vi "Z900_navX_Util_DecodeProtocol_Int8.vi"(1 "Little Endian":u8[](array[numeric])) -> (0 "Int8":i8[](array[numeric]))   [LabVIEW 2014, in "navX Library v2.lvlib"]
uses:
  navX Library v2.lvlib
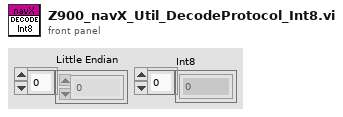
[diagram p1: front panel]
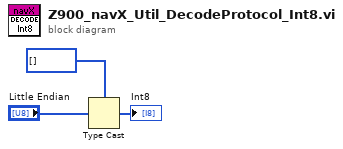
[diagram p0: block diagram]
diagram:
  n1 = Type Cast(type=i8[] [] ("Int8"), x="Little Endian") -> (*(type *) &x=→"Int8":i8[])
